vi "supress_component.vi"(6 "z":bool, 8 "error in (no error)":errorcluster, 9 "y":bool, 10 "x":bool, 11 "SpaceVector in":refnum<class "SpaceVector.lvclass">) -> (0 "error out":errorcluster, 3 "SpaceVector out":refnum<class "SpaceVector.lvclass">)   [LabVIEW 2010, in "SpaceVector.lvclass"]
uses:
  SpaceVector.lvclass
  SpaceVector.lvclass/SpaceVector.ctl
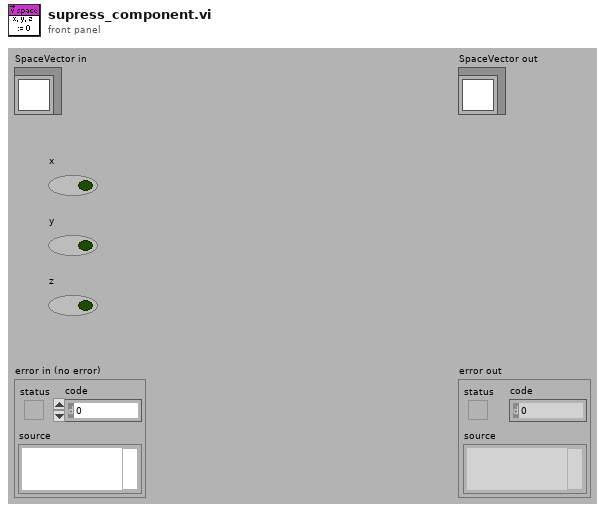
[diagram p1: front panel]
types:
  T1 = typedef "space_vector_array.ctl" = dbl[unit][]
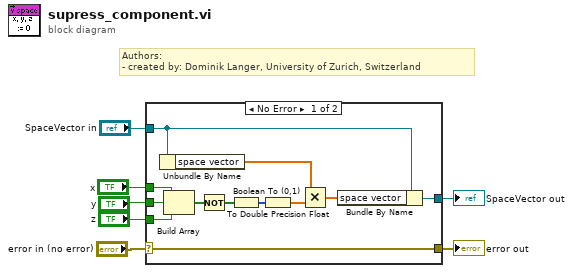
[diagram p0: block diagram]
diagram:
  # "Authors: \n- created by: Dominik Langer, University of Zurich, Switzerland"
  n1 = case shown="No Error" "error in (no error)" {
    selector: "error in (no error)" -> [w19 w21]
    tunnel: [w19 w21] -> w6
    tunnel: [w11 w20] -> w4
    tunnel: "SpaceVector in" -> [w12 w20]
    tunnel: "x" -> [w18 _]
    tunnel: "y" -> [w17 _]
    tunnel: "z" -> [w16 _]
    frame No Error {
      n2 = Unbundle By Name(w12) -> ("space vector"=w14:T1)
      n3 = Build Array(w18, w17, w16) -> (w10:bool[])
      n4 = Not(x=w10) -> (.not. x?=w9:bool[])
      n5 = Boolean To (0,1)(Boolean=w9) -> (0, 1=w15:i16[])
      n6 = To Double Precision Float(number=w15) -> (double precision float=w8:dbl[])
      n7 = Multiply(x=w14, y=w8) -> (x*y=w13:T1)
      n8 = Bundle By Name(cluster=w12, "space vector"=w13) -> (w11:refnum<class "SpaceVector.lvclass">)
    }
    frame Error {
    }
  }
  "error out" <- w6
  "SpaceVector out" <- w4
